vi "EMV Check For Increasing Temperatures.vi"(0 "Current T7 Temperatures":dbl[](array[numeric]), 1 "Detection Slope":dbl=0.2 format="%#_13g", 2 "Mixing Valve.MixValveAbsoluteStepPosition (0x400B)":i16, 5 "T7 Detection?":bool, 9 "T7_DELTA_INDICATING_FLOW":dbl, 11 "error in (no error)":errorcluster, 12 "Abnormal Input Temperature":dbl=90.0, 14 "Cold Water Supply Temperature":dbl) -> (3 "Trigger Lock":bool, 4 "Current T7 Temperatures Output":dbl[](array[numeric]), 6 "End of Flow Detection?":bool, 15 "error out":errorcluster)   [LabVIEW 2016]
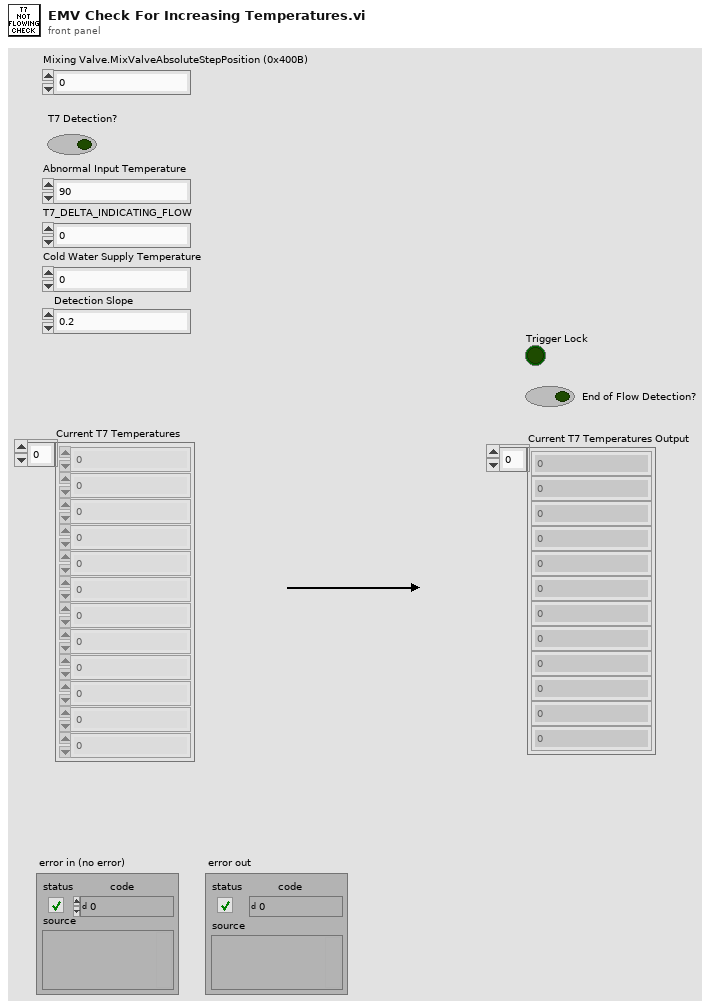
[diagram p1: front panel]
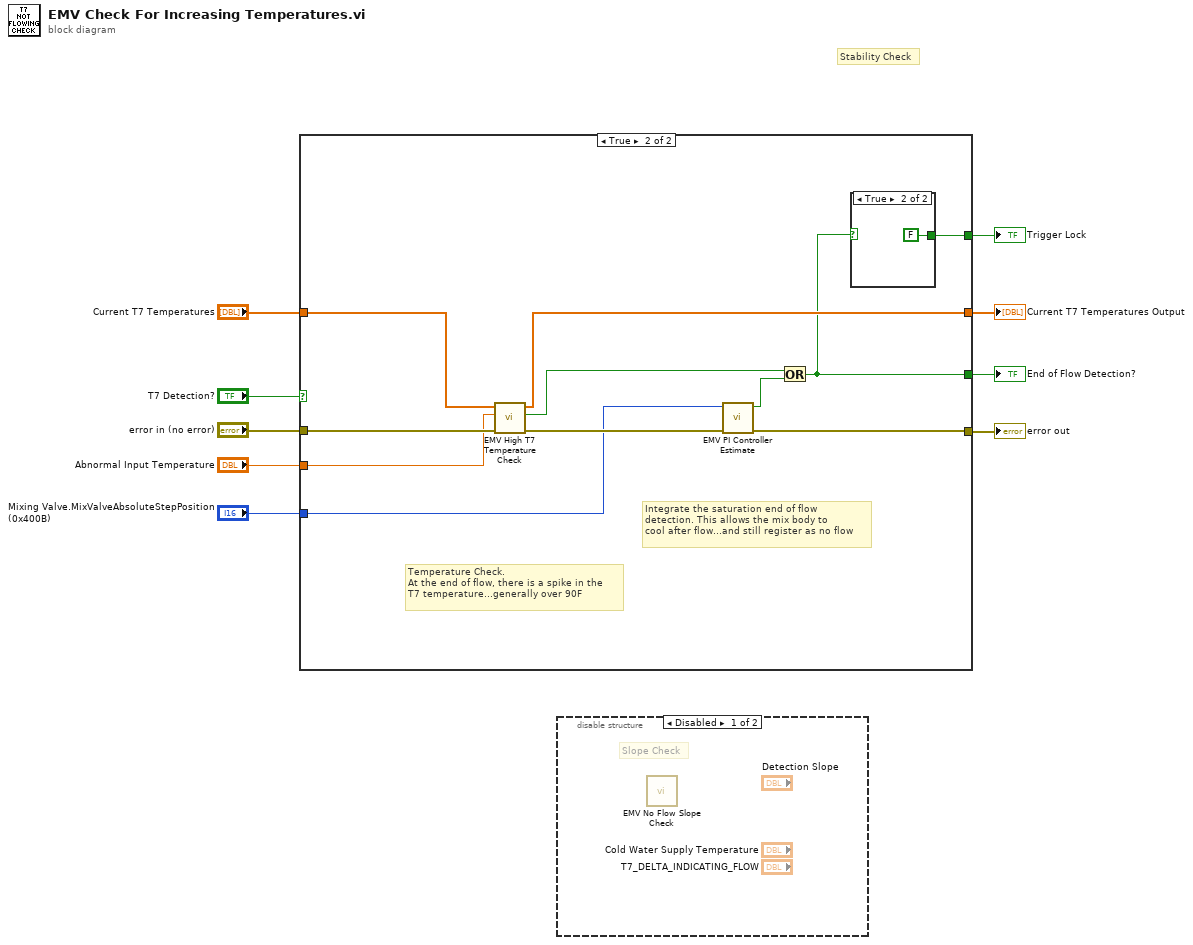
[diagram p0: block diagram]
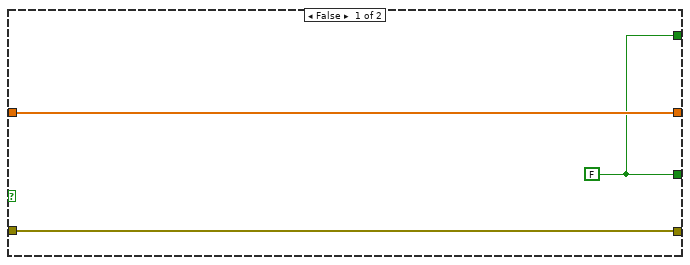
[diagram p3: hidden frame]
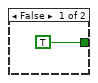
[diagram p4: hidden frame]
diagram:
  # "Stability Check"
  n1 = case shown="True" "T7 Detection?" {
    tunnel: "error in (no error)" -> [w12 w23]
    tunnel: [w10 w13] -> w7
    tunnel: [w11 w21] -> w6
    tunnel: [w12 w19] -> w5
    tunnel: "Current T7 Temperatures" -> [w11 w17]
    tunnel: "Abnormal Input Temperature" -> [_ w16]
    tunnel: "Mixing Valve.MixValveAbsoluteStepPosition (0x400B)" -> [_ w15]
    tunnel: [w10 w14] -> w1
    frame False {
      w10 = FALSE
    }
    frame True {
      # "Integrate the saturation end of flow\ndetection. This allows the mix body to \ncool after flow...and still register as no flow"
      # "Temperature Check.\nAt the end of flow, there is a spike in the \nT7 temperature...generally over 90F"
      n2 = call "EMV High T7 Temperature Check.vi"("error in (no error)"=w23, "Abnormal Input Temperature"=w16, "T7 History"=w17) -> ("error out"=w20:errorcluster, "Hot Inlet Water?"=w22:bool, "T6 History Output"=w21:dbl[])  [unwired: 6 in]
      n3 = call "EMV PI Controller Estimate.vi"("error in (no error)"=w20, "Mixing Valve.MixValveAbsoluteStepPosition (0x400B)"=w15) -> ("error out"=w19:errorcluster, "PI End of Flow Detection"=w18:bool)  [unwired: 8 in]
      n4 = Or(x=w22, y=w18) -> (x .or. y?=w13:bool)
      n5 = case shown="True" w13 {
        tunnel: [TRUE FALSE] -> w14
        frame False {
        }
        frame True {
        }
      }
    }
  }
  "End of Flow Detection?" <- w7
  "error out" <- w5
  "Current T7 Temperatures Output" <- w6
  "Trigger Lock" <- w1
  n6 = disable-structure shown="Disabled" {
    frame Disabled {
      # "Slope Check"
      n7 = call "EMV No Flow Slope Check.vi"() -> ()  [unwired: 9 in, 3 out]
    }
    frame Enabled {
    }
  }
